vi "DHE_Getrawbuffersize.vi"() -> (7 "DHE_raw_buffer_size":i32)   [LabVIEW 2016]
uses:
  private/vis/DHE_GBLDriverVariables.vi
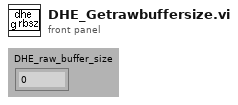
[diagram p1: front panel]
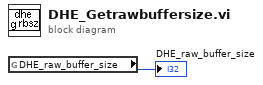
[diagram p0: block diagram]
diagram:
  n1 = global read "DHE_GBLDriverVariables.vi" "DHE_raw_buffer_size"() -> (→"DHE_raw_buffer_size":i32)
